vi "Run Continuous Digital.vi"(8 "Initialize first run":bool=TRUE, 9 "Samples / channel":i32=8192, 10 "ADALM2000 Handler":u32 caption="Instrument Handle Out") -> (2 "output waveform":digitalwaveform(waveform)={"t0"=timestamp(0 s since 1904-01-01), "dt"=1.0, "Y"={"transitions"=[], "data"=[]}}, 3 "ADALM2000 Handler 2":u32 caption="Instrument Handle Out")   [LabVIEW 2015]
uses:
  <vilib>/Waveform/DWDTOps.llb/DWDT Binary U16 to Digital.vi
  <vilib>/Waveform/DWDTOps.llb/DWDT Append Digital Samples.vi
  libm2k_lv.dll
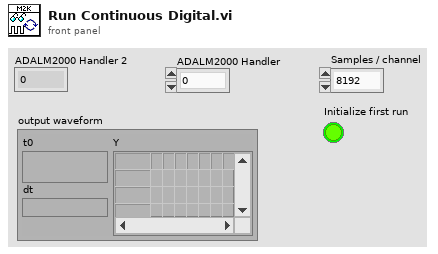
[diagram p1: front panel]
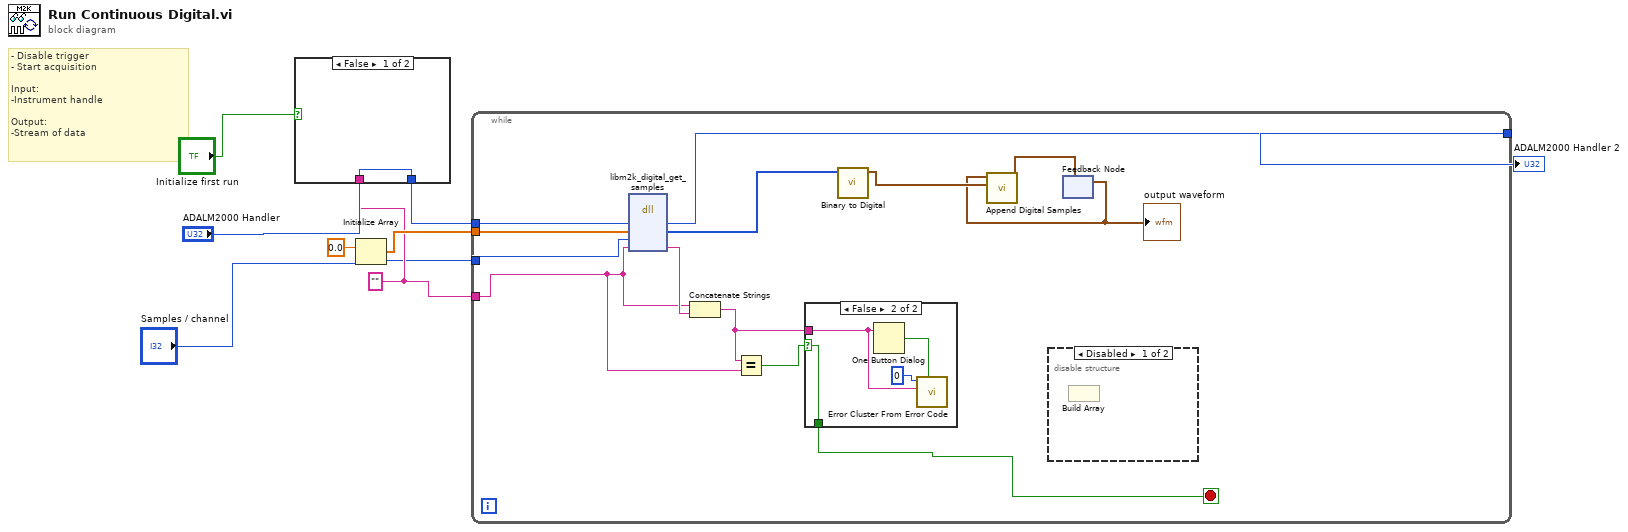
[diagram p0: block diagram]
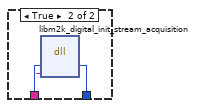
[diagram p2: hidden frame]
diagram:
  w4 = ""
  # "- Disable trigger\n- Start acquisition\n\nInput:\n-Instrument handle\n\nOutput:\n-Stream of data"
  n1 = case shown="False" "Initialize first run" {
    tunnel: "ADALM2000 Handler" -> [w9 w12]
    tunnel: [w9 w11] -> w5
    tunnel: w4 -> [_ w10]
    frame False {
    }
    frame True {
      n2 = dll-call lib="libm2k_lv.*" fn="libm2k_digital_init_stream_acquisition"("instance"=w12, "err"=w10) -> ("instance"=w11:u64)  [unwired: 5 in, 2 out]
    }
  }
  n3 = Initialize Array(0.0, "Samples / channel") -> (w7:dbl[])
  n4 = while {
    tunnel: w5 -> [w25]
    tunnel: w7 -> [w24]
    tunnel: "Samples / channel" -> [w23]
    tunnel: w4 -> [w20]
    tunnel: [w17] -> w3
    stop <- w18 stop-if-true
    n5 = dll-call lib="libm2k_lv.*" fn="libm2k_digital_get_samples"("instance"=w25, "digital_samples"=w24, "nb_samples"=w23, "err"=w20) -> ("instance"=w17:u64, "digital_samples"=w16:u16[], "err"=w22:string)  [unwired: 5 in, 2 out]
    n6 = Concatenate Strings(w20, w22) -> (w19:string)
    n7 = Equal?(x=w19, y=w20) -> (x = y?=w21:bool)
    n8 = case shown="False" w21 {
      selector: w21 -> [w26 w27]
      tunnel: w19 -> [_ w29]
      tunnel: [w26 w27] -> w18
      frame True {
      }
      frame False {
        n9 = One Button Dialog(message=w29) -> (true=w28:bool)  [unwired: 1 in]
        n10 = call <vilib>:"Error Cluster From Error Code.vi"("show call chain? (False)"=w28, "error message (\"\")"=w29, "error code (0)"=0) -> ()  [unwired: 6 in, 1 out]
      }
    }
    n11 = call-poly <vilib>:"Binary to Digital.vi"("binary array"=w16) -> ("digital waveform"=w15:digitalwaveform)  [unwired: 9 in, 1 out]
    n12 = disable-structure shown="Disabled" {
      frame Disabled {
        n13 = Build Array() -> ()  [unwired: 2 in, 1 out]
      }
      frame Enabled {
      }
    }
    n14 = feedback #1() -> (w13:digitalwaveform)  [unwired: 1 in]
    "output waveform" <- w13
    n15 = call-poly <vilib>:"Append Digital Samples.vi"("digital waveform B"=w15, "digital waveform A"=w13) -> ("digital waveform out"=w14:digitalwaveform)  [unwired: 8 in, 1 out]
    n16 = feedback-in #1(w14) -> ()
  }
  "ADALM2000 Handler 2" <- w3
